vi "Servos(SubVI).vi"() -> ()   [LabVIEW 2018]
uses:
  <vilib>/myRIO/Common/Instrument Driver Framework/myRIO v1.0/PWM/vis/myRIO v1.1 Open PWM.vi
  <vilib>/myRIO/Common/Instrument Driver Framework/myRIO v1.0/UART/vis/myRIO v1.0 Close UART.vi
  <vilib>/myRIO/Common/Instrument Driver Framework/Utilities/vis/Validate Channels.vi
  <vilib>/myRIO/Common/Instrument Driver Framework/myRIO v1.0/PWM/vis/myRIO v1.0 Reserve PWM.vi
  <vilib>/myRIO/Common/Instrument Driver Framework/myRIO v1.0/PWM/vis/myRIO v1.0 Build MUX Configuration PWM.vi
  <vilib>/myRIO/Common/Instrument Driver Framework/myRIO v1.0/Resource Manager/vis/myRIO v1.0 Reserve Channel List.vi
  <vilib>/myRIO/Common/Instrument Driver Framework/myRIO v1.0/Resource Manager/vis/myRIO v1.0 Create Configuration List.vi
  <vilib>/myRIO/Common/Instrument Driver Framework/myRIO v1.0/Resource Manager/vis/myRIO v1.0 Reserve Channel.vi
  <vilib>/myRIO/Common/Instrument Driver Framework/myRIO v1.0/Resource Manager/vis/myRIO v1.0 Unreserve Channel.vi
  <vilib>/myRIO/Common/Instrument Driver Framework/myRIO v1.0/Resource Manager/vis/myRIO v1.0 Build Mutex Name.vi
  <vilib>/Utility/VariantDataType/GetNumericInfo.vi
  <vilib>/Utility/error.llb/Error Cluster From Error Code.vi
  <vilib>/myRIO/Common/Instrument Driver Framework/myRIO v1.0/myRIO v1.1 Open.vi
  <vilib>/myRIO/Common/Instrument Driver Framework/Utilities/vis/IO Manager.vi
  <vilib>/myRIO/Common/Instrument Driver Framework/Utilities/vis/Configuration Manager.vi
  <vilib>/myRIO/Common/Instrument Driver Framework/myRIO v1.0/Resource Manager/vis/myRIO v1.0 Configure IO.vi
  <vilib>/myRIO/Common/Instrument Driver Framework/myRIO v1.0/myRIO v1.0 Close.vi
  <vilib>/myRIO/Common/Instrument Driver Framework/myRIO v1.0/PWM/vis/myRIO v1.0 Write PWM.vi
  <vilib>/myRIO/Common/Instrument Driver Framework/Utilities/vis/FPGA Ref Manager.vi
  <vilib>/myRIO/Common/Instrument Driver Framework/myRIO v1.0/myRIO v1.0 Reset FPGA.vi
  <vilib>/myRIO/Common/Instrument Driver Framework/myRIO v1.0/IRQ/vis/myRIO v1.0 IRQ Info FGV.vi
  <vilib>/myRIO/Common/Instrument Driver Framework/myRIO v1.0/IRQ/vis/myRIO v1.0 Timer IRQ Info FGV.vi
  <vilib>/myRIO/Common/Instrument Driver Framework/myRIO v1.0/IRQ/vis/myRIO v1.0 ISR Agent.vi
  <vilib>/myRIO/Instrument Drivers/Utilities/Utilities.lvlib
  <vilib>/myRIO/Instrument Drivers/Onboard IO/PWM/PWM.lvlib
panel:
  in  "Second":dbl(slide) scale=-200.0..200.0
  in  "freq [Hz] 2":dbl=50.0
  out "pulse width [ms] 2":dbl=1.5
  out "duty cycle [%] 2":dbl
  in  "null offset 2":bool
  out "offset [%FS] 2":dbl
  in  "[ESC]":bool
  in  "First":dbl(slide) min=-500.0 scale=-200.0..200.0
  in  "freq [Hz]":dbl=50.0
  out "pulse width [ms]":dbl=1.5
  out "duty cycle [%]":dbl
  in  "null offset":bool
  out "offset [%FS]":dbl
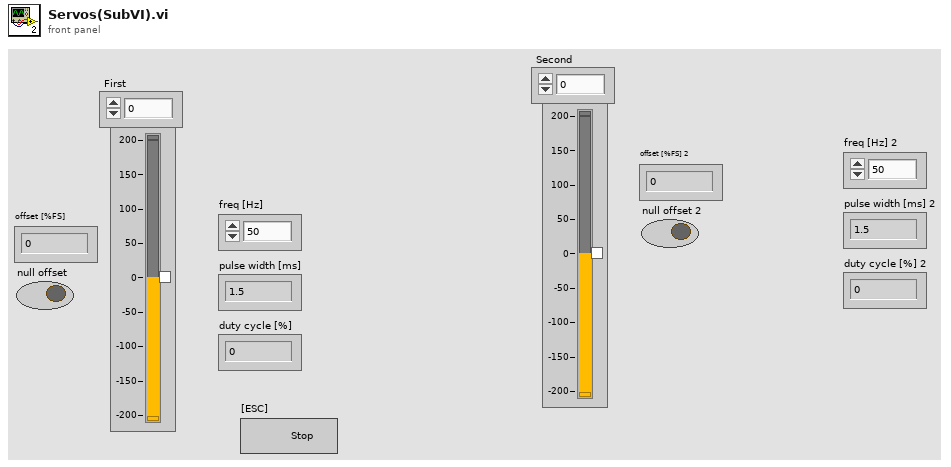
[diagram p1: front panel]
types:
  T1 = typedef "PWM.lvlib/PWM Reference.ctl" = cluster{"myRIO Reference":T2, "PWM Channels Enum":T6, "PWM Configuration":T7}
  T2 = typedef "myRIO Generic Hardware Reference.ctl" = cluster{"myRIO Model":T3, "myRIO Hardware Reference":T4}
  T3 = typedef "Hardware Version Enum.ctl" = enum16{"Unknown", "myRIO-1900", "myRIO-1950", "roboRIO", "NI ELVIS RIO CM", "ELVIS III"}
  T4 = typedef "myRIO v1.0 Reference.ctl" = cluster{"Generic FPGA Reference":T5, "Allow multiple opens":bool}
  T5 = typedef "Generic FPGA Reference.ctl" = refnum<k20>
  T6 = typedef "PWM Channels Enum.ctl" = enum16{"Not Connected", "C/PWM0", "C/PWM1", "A/PWM0", "A/PWM1", "A/PWM2", "A/PWM3", "A/PWM4", "A/PWM5", "A/PWM6", "A/PWM7", "A/PWM8", "A/PWM9", "A/PWM10", "A/PWM11", "A/PWM12", "A/PWM13", "A/PWM14", "A/PWM15", "A/PWM16", "A/PWM17", "A/PWM18", "A/PWM19", "B/PWM0", "B/PWM1", "B/PWM2", "B/PWM3", "B/PWM4", "B/PWM5", "B/PWM6", "B/PWM7", "B/PWM8", "B/PWM9", "B/PWM10", "B/PWM11", "B/PWM12", "B/PWM13", "B/PWM14", "B/PWM15", "B/PWM16", "B/PWM17", "B/PWM18", "B/PWM19", "PWM/PWM0", "PWM/PWM1", "PWM/PWM2", "PWM/PWM3", "PWM/PWM4", "PWM/PWM5", "PWM/PWM6", "PWM/PWM7", "PWM/PWM8", "PWM/PWM9"}
  T7 = typedef "PWM.lvlib/PWM Configuration.ctl" = cluster{"Frequency":dbl, "Duty Cycle":dbl}
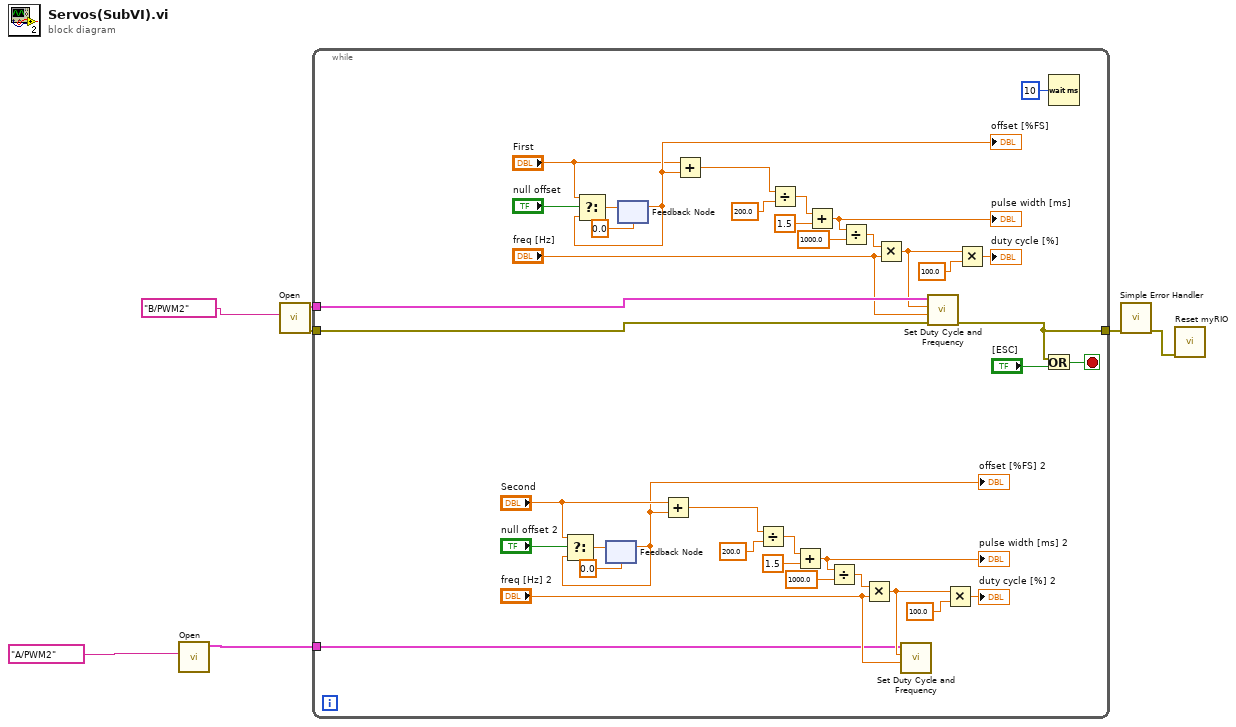
[diagram p0: block diagram]
diagram:
  n1 = call <vilib>:"Open.vi"("Channel Name"=tag "A/PWM2" ("PWM channel 2")) -> ("PWM Ref Out"=w1:T1)  [unwired: 9 in, 1 out]
  n2 = call <vilib>:"Open.vi"("Channel Name"=tag "B/PWM2" ("PWM channel")) -> ("error out"=w4:errorcluster, "PWM Ref Out"=w5:T1)  [unwired: 9 in]
  n3 = while {
    tunnel: w5 -> [w38]
    tunnel: w4 -> [w37]
    tunnel: [w35] -> w3
    tunnel: w1 -> [w8]
    stop <- w46 stop-if-true
    n4 = feedback #1(0.0 ("position [%FS]")) -> (w20:dbl)
    "offset [%FS] 2" <- w20
    n5 = Select(t="Second", s="null offset 2", f=w20) -> (s? t:f=w9:dbl)
    n6 = feedback-in #1(w9) -> ()
    n7 = feedback #2(0.0 ("position [%FS]")) -> (w31:dbl)
    "offset [%FS]" <- w31
    n8 = Select(t="First", s="null offset", f=w31) -> (s? t:f=w33:dbl)
    n9 = feedback-in #2(w33) -> ()
    n10 = Add(x="Second", y=w20) -> (x+y=w19:dbl)
    n11 = Add(x="First", y=w31) -> (x+y=w32:dbl)
    n12 = Divide(x=w19, y=200.0) -> (x/y=w15:dbl)
    n13 = Divide(x=w32, y=200.0) -> (x/y=w42:dbl)
    n14 = Add(x=w15, y=1.5) -> (x+y=w16:dbl)
    "pulse width [ms] 2" <- w16
    n15 = Add(x=w42, y=1.5) -> (x+y=w40:dbl)
    "pulse width [ms]" <- w40
    n16 = Divide(x=w16, y=1000.0) -> (x/y=w22:dbl)
    n17 = Divide(x=w40, y=1000.0) -> (x/y=w29:dbl)
    n18 = Multiply(x=w22, y="freq [Hz] 2") -> (x*y=w24:dbl)
    n19 = Multiply(x=w29, y="freq [Hz]") -> (x*y=w26:dbl)
    n20 = call <vilib>:"Set Duty Cycle and Frequency.vi"("Frequency [Hz]"="freq [Hz] 2", "Duty Cycle"=w24, "PWM Ref In"=w8) -> ()  [unwired: 6 in, 2 out]
    n21 = call <vilib>:"Set Duty Cycle and Frequency.vi"("error in (no error)"=w37, "Frequency [Hz]"="freq [Hz]", "Duty Cycle"=w26, "PWM Ref In"=w38) -> ("error out"=w35:errorcluster)  [unwired: 5 in, 1 out]
    n22 = Multiply(x=w24, y=100.0) -> (x*y=→"duty cycle [%] 2":dbl)
    n23 = Multiply(x=w26, y=100.0) -> (x*y=→"duty cycle [%]":dbl)
    n24 = Or(x=w35, y="[ESC]") -> (x .or. y?=w46:bool)
    n25 = Wait (ms)(milliseconds to wait=u32 10) -> ()  [unwired: 1 out]
  }
  n26 = call <vilib>:"Simple Error Handler.vi"("error in (no error)"=w3) -> ("error out"=w7:errorcluster)  [unwired: 4 in, 4 out]
  n27 = call <vilib>:"Reset myRIO.vi"("error in (no error)"=w7) -> ()  [unwired: 10 in, 1 out]
